vi "Read Home State.vi"(8 "error in (no error)":errorcluster, 11 "Filter Wheel in":refnum<class "Filter Wheel.lvclass">) -> (0 "error out":errorcluster, 2 "Home State":bool[](array[boolean]), 3 "Filter Wheel out":refnum<class "Filter Wheel.lvclass">)   [LabVIEW 2021, in "Filter Wheel.lvclass"]
uses:
  Filter Wheel.lvclass
  Filter Wheel.lvclass/Filter Wheel.ctl
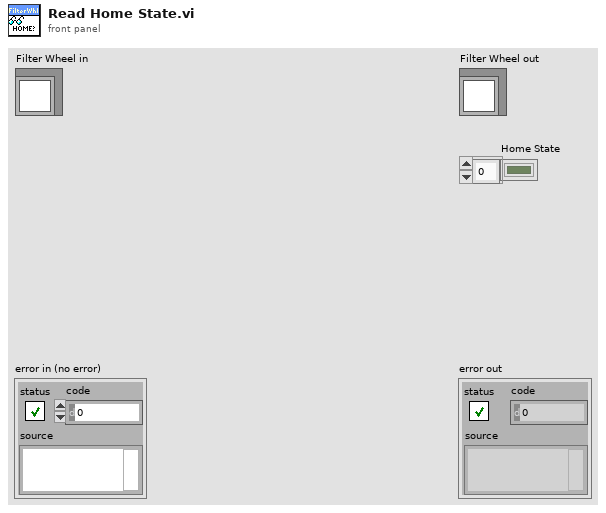
[diagram p1: front panel]
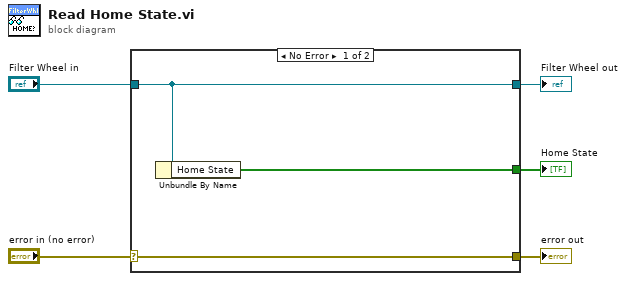
[diagram p0: block diagram]
diagram:
  n1 = case shown="No Error" "error in (no error)" {
    selector: "error in (no error)" -> [w8 w9]
    tunnel: [w8 w9] -> w4
    tunnel: [w7 w10] -> w2
    tunnel: "Filter Wheel in" -> [w7 w10]
    tunnel: [w6 _] -> w1
    frame No Error {
      n2 = Unbundle By Name(w7) -> ("Home State"=w6:bool[])
    }
    frame Error {
    }
  }
  "error out" <- w4
  "Filter Wheel out" <- w2
  "Home State" <- w1
